vi "populate available tags.vi"(7 "instance id":string, 8 "error in":errorcluster, 9 "channel":refnum<class "TBM channel.lvclass">, 10 "CtlRef":refnum<vi>, 11 "engine configuration in":refnum<class "engine configuration.lvclass">) -> (0 "error out":errorcluster, 3 "engine configuration out":refnum<class "engine configuration.lvclass">)   [LabVIEW 2013, in "user tag bus module editor node.lvclass"]
uses:
  user tag bus module editor node.lvclass
  <vilib>/NI/Tag Bus Module Framework/channel/TBM channel.lvclass
  <vilib>/NI/Module Execution Interface/Engine Configuration/engine configuration.lvclass
  <vilib>/NI/Tag Bus Module Framework/channel/TBM channel.lvclass/TBM channel.ctl
  <vilib>/NI/Tag Bus/tag/tag descriptor.lvclass
  <vilib>/NI/Tag Bus/tag/tag descriptor.lvclass/tag descriptor.ctl
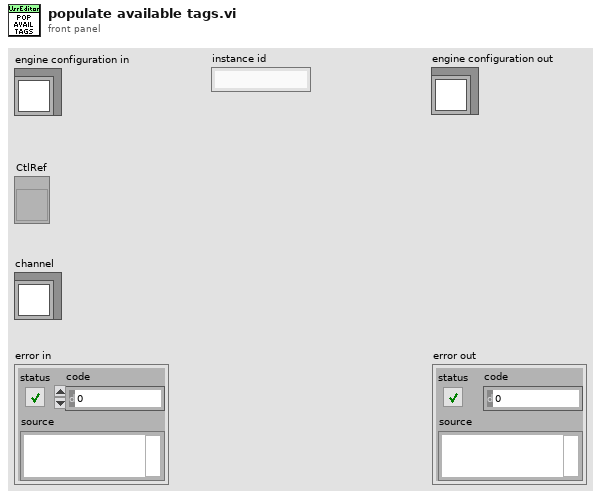
[diagram p1: front panel]
types:
  T1 = typedef "TBM channel.lvclass/channel classification.ctl" = enum16{"input data", "output data", "processing parameter", "processing result"}
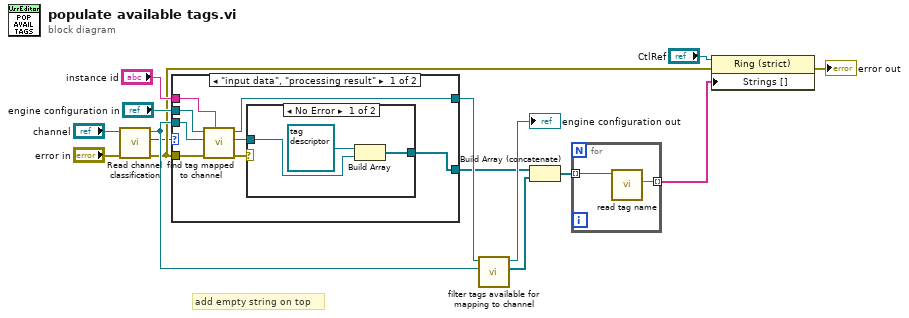
[diagram p0: block diagram]
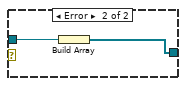
[diagram p2: hidden frame]
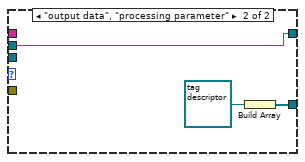
[diagram p3: hidden frame]
diagram:
  # "add empty string on top"
  n1 = call <vilib>:"Read channel classification.vi"("error in"="error in", "channel in"="channel") -> ("error out"=w2:errorcluster, "channel classification"=w1:T1, "channel out"=w4:refnum<class "TBM channel.lvclass">)  [unwired: 7 in]
  n2 = case shown="\"input data\", \"processing result\"" w1 {
    tunnel: "instance id" -> [w23 _]
    tunnel: [w22 w29] -> w14
    tunnel: "engine configuration in" -> [w21 w29]
    tunnel: [w18 w30] -> w6
    tunnel: w4 -> [w17 _]
    tunnel: w2 -> [w16 _]
    frame "input data", "processing result" {
      n3 = call <vilib>:"find tag mapped to channel.vi"("owner"=w23, "error in"=w16, "channel"=w17, "engine configuration in"=w21) -> ("error out"=w20:errorcluster, "tag"=w19:refnum<class "tag descriptor.lvclass">, "engine configuration out"=w22:refnum<class "engine configuration.lvclass">)  [unwired: 5 in]
      n4 = case shown="No Error" w20 {
        tunnel: w19 -> [w26 w27]
        tunnel: [w24 w28] -> w18
        frame No Error {
          n5 = Build Array(refnum<class "tag descriptor.lvclass"> refnum ("tag"), w26) -> (w24:refnum<class "tag descriptor.lvclass">[])
        }
        frame Error {
          n6 = Build Array(w27) -> (w28:refnum<class "tag descriptor.lvclass">[])
        }
      }
    }
    frame "output data", "processing parameter" {
      n7 = Build Array(refnum<class "tag descriptor.lvclass"> refnum ("tag")) -> (w30:refnum<class "tag descriptor.lvclass">[])
    }
  }
  n8 = call <vilib>:"filter tags available for mapping to channel.vi"("channel to map to"=w4, "engine configuration in"=w14) -> ("filtered tags"=w8:refnum<class "tag descriptor.lvclass">[], "engine configuration out"=→"engine configuration out":refnum<class "engine configuration.lvclass">)  [unwired: 8 in]
  n9 = Build Array (concatenate)(w6, w8) -> (w9:refnum<class "tag descriptor.lvclass">[])
  n10 = for {
    tunnel: w9 -> [w32] mode=indexing
    tunnel: [w33] -> w11 mode=indexing
    n11 = call <vilib>:"read tag name.vi"("system tag in"=w32) -> ("name"=w33:string)  [unwired: 8 in, 2 out]
  }
  n12 = property on="Property Node" class="Ring (strict)"(reference="CtlRef", error in=w2, "Strings []"=w11) -> (error out=→"error out":errorcluster)  [unwired: 1 out]
